vi "输入数据解析.vi"(0 "单个参数补充":dbl, 1 "从板号":dbl=1.0, 2 "主板二维码":string="BNET01", 3 "从板二维码":string="BNET01", 5 "主板引用":refnum<vi>, 7 "从板引用":refnum<vi>, 9 "主板选项":string="三级故障阀值", 11 "枚举":enum16{"主板", "从板"}(ring), 12 "快换":bool caption="快换写入") -> (4 "输出数组":dbl[][](array[numeric]), 6 "数组长度":dbl[](array[numeric]), 8 "循环次数":i32, 10 "命令":u32, 14 "名称":string[](array[string]), 15 "命令序号":u32[](array[numeric]))   [LabVIEW 2013] (continued)
                    n2574 = call "输入分辨率计算-EV05.vi"("1字节?"=FALSE, "数值"=w6626, "偏移量"=0.0, "分辨率"=0.001) -> ("低字节"=w6628:dbl, "高字节1"=w6630:dbl)  [unwired: 1 in, 5 out]
                  }
                  frame Enabled {
                    w6633 = 255 ("高字节1")
                  }
                }
                n2575 = Build Array(w6625, w6623) -> (w6624:i32[])
              }
              frame 7 {
                # "单体电压过高"
                n2576 = disable-structure shown="启用" {
                  disable-tunnel: [w6642 w6645] -> w6637
                  disable-tunnel: [w6640 w6645] -> w6635
                  disable-tunnel: w6634 -> [w6639 _]
                  frame Disabled {
                    n2577 = Unbundle By Name(w6639) -> ("单体电压过高"=w6638:dbl)
                    n2578 = call "输入分辨率计算-EV05.vi"("1字节?"=FALSE, "数值"=w6638, "偏移量"=0.0, "分辨率"=0.001) -> ("低字节"=w6640:dbl, "高字节1"=w6642:dbl)  [unwired: 1 in, 5 out]
                  }
                  frame Enabled {
                    w6645 = 255 ("高字节1")
                  }
                }
                n2579 = Build Array(w6637, w6635) -> (w6636:i32[])
              }
              frame 8 {
                # "单体电压过低"
                n2580 = disable-structure shown="启用" {
                  disable-tunnel: [w6654 w6657] -> w6649
                  disable-tunnel: [w6652 w6657] -> w6647
                  disable-tunnel: w6646 -> [w6651 _]
                  frame Enabled {
                    n2581 = Unbundle By Name(w6651) -> ("单体电压过低"=w6650:dbl)
                    n2582 = call "输入分辨率计算-EV05.vi"("1字节?"=FALSE, "数值"=w6650, "偏移量"=0.0, "分辨率"=0.001) -> ("低字节"=w6652:dbl, "高字节1"=w6654:dbl)  [unwired: 1 in, 5 out]
                  }
                  frame Disabled {
                    w6657 = 255 ("高字节1")
                  }
                }
                n2583 = Build Array(w6649, w6647) -> (w6648:dbl[])
              }
              frame 9 {
                # "充电电流过高"
                n2584 = disable-structure shown="启用" {
                  disable-tunnel: [w6666 w6669] -> w6661
                  disable-tunnel: [w6664 w6669] -> w6659
                  disable-tunnel: w6658 -> [w6663 _]
                  frame Disabled {
                    n2585 = Unbundle By Name(w6663) -> ("充电电流过高"=w6662:dbl)
                    n2586 = call "输入分辨率计算-EV05.vi"("1字节?"=FALSE, "数值"=w6662, "偏移量"=-3000.0, "分辨率"=0.1) -> ("低字节"=w6664:dbl, "高字节1"=w6666:dbl)  [unwired: 1 in, 5 out]
                  }
                  frame Enabled {
                    w6669 = 255 ("高字节1")
                  }
                }
                n2587 = Build Array(w6661, w6659) -> (w6660:i32[])
              }
              frame 10 {
                # "放电电流过高"
                n2588 = disable-structure shown="启用" {
                  disable-tunnel: [w6678 w6681] -> w6673
                  disable-tunnel: [w6676 w6681] -> w6671
                  disable-tunnel: w6670 -> [w6675 _]
                  frame Disabled {
                    n2589 = Unbundle By Name(w6675) -> ("放电电流过高"=w6674:dbl)
                    n2590 = call "输入分辨率计算-EV05.vi"("1字节?"=FALSE, "数值"=w6674, "偏移量"=-3000.0, "分辨率"=0.1) -> ("低字节"=w6676:dbl, "高字节1"=w6678:dbl)  [unwired: 1 in, 5 out]
                  }
                  frame Enabled {
                    w6681 = 255 ("高字节1")
                  }
                }
                n2591 = Build Array(w6673, w6671) -> (w6672:i32[])
              }
              frame 11 {
                # "单组温度不均衡"
                n2592 = disable-structure shown="启用" {
                  disable-tunnel: [w6688 255 ("高字节1")] -> w6684
                  disable-tunnel: w6682 -> [w6686 _]
                  frame Disabled {
                    n2593 = Unbundle By Name(w6686) -> ("单组温度不均衡"=w6685:dbl)
                    n2594 = call "输入分辨率计算-EV05.vi"("1字节?"=TRUE, "数值"=w6685, "偏移量"=0.0, "分辨率"=1.0) -> ("高字节1"=w6688:dbl)  [unwired: 1 in, 6 out]
                  }
                  frame Enabled {
                  }
                }
                n2595 = Build Array(w6684) -> (w6683:i32[])
              }
              frame 12 {
                # "SOC过高"
                n2596 = Unbundle By Name(w6696) -> ("SOC过高"=w6695:dbl)
                n2597 = call "输入分辨率计算-EV05.vi"("1字节?"=FALSE, "数值"=w6695, "偏移量"=0.0, "分辨率"=0.1) -> ("低字节"=w6697:dbl, "高字节1"=w6698:dbl)  [unwired: 1 in, 5 out]
                n2598 = call "二进制解析-8.6.vi"("索引"=4, "数值"=w6698) -> ("低位子数组"=w6701:i32[])  [unwired: 3 out]
                n2599 = call "二进制解析-8.6.vi"("索引"=4, "数值"=w6697) -> ("低位子数组"=w6693:i32[], "高位子数组"=w6700:i32[])  [unwired: 2 out]
                n2600 = Insert Into Array(array=w6701, new element=w6700) -> (w6699:i32[])  [unwired: 1 in]
                n2601 = call "数值二进制转十进制-8.6.vi"("子数组"=w6699) -> ("十进制数值"=w6694:i32)  [unwired: 4 out]
                n2602 = disable-structure shown="启用" {
                  disable-tunnel: w6694 -> [w6709 _]
                  disable-tunnel: [w6709 255 ("高字节1")] -> w6692
                  disable-tunnel: [w6708 i32[] [] ("低位子数组 26")] -> _
                  disable-tunnel: w6693 -> [w6708 _]
                  frame Disabled {
                  }
                  frame Enabled {
                  }
                }
                n2603 = Build Array(w6692, w6692) -> (w6705:i32[])
              }
              frame 13 {
                # "SOC过低"
                n2604 = Unbundle By Name(w6717) -> ("SOC过低"=w6716:dbl)
                n2605 = call "输入分辨率计算-EV05.vi"("1字节?"=FALSE, "数值"=w6716, "偏移量"=0.0, "分辨率"=0.1) -> ("低字节"=w6714:dbl, "高字节1"=w6715:dbl)  [unwired: 1 in, 5 out]
                n2606 = call "二进制解析-8.6.vi"("索引"=4, "数值"=w6715) -> ("低位子数组"=w6713:i32[])  [unwired: 3 out]
                n2607 = disable-structure shown="启用" {
                  disable-tunnel: w6714 -> [w6724 _]
                  disable-tunnel: [w6724 255 ("高字节1")] -> w6712
                  disable-tunnel: w6713 -> [w6723 _]
                  frame Disabled {
                    (unwired) i32[] [] ("低位子数组 4")
                  }
                  frame Enabled {
                  }
                }
                n2608 = Build Array(w6712, w6712) -> (w6720:i32[])
              }
              frame 14 {
                # "内阻过大"
                n2609 = disable-structure shown="启用" {
                  disable-tunnel: w6728 -> [w6733 _]
                  disable-tunnel: [w6729 255 ("高字节1")] -> w6726
                  frame Disabled {
                    n2610 = Unbundle By Name(w6733) -> ("内阻过大"=w6732:dbl)
                    n2611 = call "输入分辨率计算-EV05.vi"("1字节?"=TRUE, "数值"=w6732, "分辨率"=0.1) -> ("高字节1"=w6729:dbl)  [unwired: 2 in, 6 out]
                  }
                  frame Enabled {
                  }
                }
                n2612 = Build Array(w6726) -> (w6727:i32[])
              }
              frame 15 {
                # "极柱温度过高"
                n2613 = disable-structure shown="启用" {
                  disable-tunnel: w6737 -> [w6743 _]
                  disable-tunnel: [w6739 255 ("高字节1")] -> w6735
                  frame Disabled {
                    n2614 = Unbundle By Name(w6743) -> ("极柱温度过高"=w6742:dbl)
                    n2615 = call "输入分辨率计算-EV05.vi"("1字节?"=TRUE, "数值"=w6742, "偏移量"=-40.0, "分辨率"=1.0) -> ("高字节1"=w6739:dbl)  [unwired: 1 in, 6 out]
                  }
                  frame Enabled {
                  }
                }
                n2616 = Build Array(w6735) -> (w6736:i32[])
              }
              frame 16 {
                # "SOH过低"
                n2617 = disable-structure shown="启用" {
                  disable-tunnel: [w6760 w6768] -> w6747
                  disable-tunnel: w6746 -> [w6757 _]
                  disable-tunnel: [w6749 w6768] -> w6745
                  frame Disabled {
                    n2618 = Unbundle By Name(w6757) -> ("SOH过低"=w6756:dbl)
                    n2619 = call "输入分辨率计算-EV05.vi"("1字节?"=FALSE, "数值"=w6756, "偏移量"=0.0, "分辨率"=0.1) -> ("低字节"=w6758:dbl, "高字节1"=w6759:dbl)  [unwired: 1 in, 5 out]
                    n2620 = call "二进制解析-8.6.vi"("索引"=4, "数值"=w6759) -> ("低位子数组"=w6762:i32[])  [unwired: 3 out]
                    n2621 = call "二进制解析-8.6.vi"("索引"=4, "数值"=w6758) -> ("低位子数组"=w6751:i32[], "高位子数组"=w6761:i32[])  [unwired: 2 out]
                    n2622 = call "二进制解析-8.6.vi"("索引"=4, "数值"=0) -> ("低位子数组"=w6752:i32[])  [unwired: 3 out]
                    n2623 = Insert Into Array(array=w6762, new element=w6761) -> (w6755:i32[])  [unwired: 1 in]
                    n2624 = Insert Into Array(array=w6751, new element=w6752) -> (w6750:i32[])  [unwired: 1 in]
                    n2625 = call "数值二进制转十进制-8.6.vi"("子数组"=w6755) -> ("十进制数值"=w6760:i32)  [unwired: 4 out]
                    n2626 = call "数值二进制转十进制-8.6.vi"("子数组"=w6750) -> ("十进制数值"=w6749:i32)  [unwired: 4 out]
                  }
                  frame Enabled {
                    w6768 = 255 ("高字节1")
                  }
                }
                n2627 = Build Array(w6747, w6745) -> (w6748:i32[])
              }
            }
            n2628 = Insert Into Array(array=w6554, new element=w6555) -> (w6553:dbl[])  [unwired: 1 in]
          }
          n2629 = Build Array(w6550) -> (w6549:dbl[][])
          n2630 = Build Array("一级故障阀值") -> (w6540:string[])
        }
        frame "单体电压过低(2)" {
          n2631 = Unbundle By Name(w6774) -> ("一级故障 2"=w6775:refnum<vi>)
          n2632 = property class="Clust (严格)"(reference=w6775) -> ("Value"=w6773:T4)  [unwired: 1 in, 2 out]
          n2633 = for {
            N: 17 -> [_]
            tunnel: w6773 -> [w6785]
            shift-right: [w6782] -> w6779
            shift-left: dbl[] [] -> [w6783]
            i -> [w6786]
            n2634 = case shown="13" w6786 {
              tunnel: w6785 -> [w6787 w6798 w6809 w6819 w6829 w6839 w6851 w6863 w6875 w6887 w6899 w6911 w6925 w6946 w6957 w6966 w6975]
              tunnel: [w6788 w6799 w6810 w6820 w6830 w6841 w6853 w6865 w6877 w6889 w6901 w6912 w6934 w6949 w6956 w6965 w6977] -> w6784
              frame 0, Default {
                # "总电压过高"
                n2635 = disable-structure shown="启用" {
                  disable-tunnel: [w6794 w6797] -> w6790
                  disable-tunnel: [w6793 w6797] -> w6789
                  disable-tunnel: w6787 -> [w6792 _]
                  frame Disabled {
                    n2636 = Unbundle By Name(w6792) -> ("总电压过高"=w6791:dbl)
                    n2637 = call "输入分辨率计算-EV05.vi"("1字节?"=FALSE, "数值"=w6791, "分辨率"=0.1) -> ("低字节"=w6794:dbl, "高字节1"=w6793:dbl)  [unwired: 2 in, 5 out]
                  }
                  frame Enabled {
                    w6797 = 255 ("高字节1")
                  }
                }
                n2638 = Build Array(w6789, w6790) -> (w6788:i32[])
              }
              frame 1 {
                # "总电压过低"
                n2639 = disable-structure shown="启用" {
                  disable-tunnel: [w6805 w6808] -> w6801
                  disable-tunnel: [w6804 w6808] -> w6800
                  disable-tunnel: w6798 -> [w6803 _]
                  frame Disabled {
                    n2640 = Unbundle By Name(w6803) -> ("总电压过低"=w6802:dbl)
                    n2641 = call "输入分辨率计算-EV05.vi"("1字节?"=FALSE, "数值"=w6802, "分辨率"=0.1) -> ("低字节"=w6805:dbl, "高字节1"=w6804:dbl)  [unwired: 2 in, 5 out]
                  }
                  frame Enabled {
                    w6808 = 255 ("高字节1")
                  }
                }
                n2642 = Build Array(w6800, w6801) -> (w6799:i32[])
              }
              frame 2 {
                # "温度过高"
                n2643 = disable-structure shown="启用" {
                  disable-tunnel: [w6815 255 ("高字节1")] -> w6811
                  disable-tunnel: w6809 -> [w6813 _]
                  frame Disabled {
                    n2644 = Unbundle By Name(w6813) -> ("温度过高"=w6812:dbl)
                    n2645 = call "输入分辨率计算-EV05.vi"("1字节?"=TRUE, "数值"=w6812, "偏移量"=-40.0, "分辨率"=1.0) -> ("高字节1"=w6815:dbl)  [unwired: 1 in, 6 out]
                  }
                  frame Enabled {
                  }
                }
                n2646 = Build Array(w6811) -> (w6810:i32[])
              }
              frame 3 {
                # "温度过低"
                n2647 = disable-structure shown="启用" {
                  disable-tunnel: [w6825 255 ("高字节1")] -> w6821
                  disable-tunnel: w6819 -> [w6823 _]
                  frame Disabled {
                    n2648 = Unbundle By Name(w6823) -> ("温度过低"=w6822:dbl)
                    n2649 = call "输入分辨率计算-EV05.vi"("1字节?"=TRUE, "数值"=w6822, "偏移量"=-40.0, "分辨率"=1.0) -> ("高字节1"=w6825:dbl)  [unwired: 1 in, 6 out]
                  }
                  frame Enabled {
                  }
                }
                n2650 = Build Array(w6821) -> (w6820:i32[])
              }
              frame 4 {
                # "整组温度不均衡"
                n2651 = disable-structure shown="启用" {
                  disable-tunnel: [w6835 255 ("高字节1")] -> w6831
                  disable-tunnel: w6829 -> [w6833 _]
                  frame Disabled {
                    n2652 = Unbundle By Name(w6833) -> ("整组温度不均衡"=w6832:dbl)
                    n2653 = call "输入分辨率计算-EV05.vi"("1字节?"=TRUE, "数值"=w6832, "偏移量"=0.0, "分辨率"=1.0) -> ("高字节1"=w6835:dbl)  [unwired: 1 in, 6 out]
                  }
                  frame Enabled {
                  }
                }
                n2654 = Build Array(w6831) -> (w6830:i32[])
              }
              frame 5 {
                # "单组电压不均衡"
                n2655 = disable-structure shown="启用" {
                  disable-tunnel: [w6847 w6850] -> w6842
                  disable-tunnel: [w6845 w6850] -> w6840
                  disable-tunnel: w6839 -> [w6844 _]
                  frame Disabled {
                    n2656 = Unbundle By Name(w6844) -> ("单组电压不均衡"=w6843:dbl)
                    n2657 = call "输入分辨率计算-EV05.vi"("1字节?"=FALSE, "数值"=w6843, "偏移量"=0.0, "分辨率"=0.001) -> ("低字节"=w6845:dbl, "高字节1"=w6847:dbl)  [unwired: 1 in, 5 out]
                  }
                  frame Enabled {
                    w6850 = 255 ("高字节1")
                  }
                }
                n2658 = Build Array(w6842, w6840) -> (w6841:i32[])
              }
              frame 6 {
                # "整组电压不均衡"
                n2659 = disable-structure shown="启用" {
                  disable-tunnel: [w6859 w6862] -> w6854
                  disable-tunnel: [w6857 w6862] -> w6852
                  disable-tunnel: w6851 -> [w6856 _]
                  frame Disabled {
                    n2660 = Unbundle By Name(w6856) -> ("整组电压不均衡"=w6855:dbl)
                    n2661 = call "输入分辨率计算-EV05.vi"("1字节?"=FALSE, "数值"=w6855, "偏移量"=0.0, "分辨率"=0.001) -> ("低字节"=w6857:dbl, "高字节1"=w6859:dbl)  [unwired: 1 in, 5 out]
                  }
                  frame Enabled {
                    w6862 = 255 ("高字节1")
                  }
                }
                n2662 = Build Array(w6854, w6852) -> (w6853:i32[])
              }
              frame 7 {
                # "单体电压过高"
                n2663 = disable-structure shown="启用" {
                  disable-tunnel: [w6871 w6874] -> w6866
                  disable-tunnel: [w6869 w6874] -> w6864
                  disable-tunnel: w6863 -> [w6868 _]
                  frame Disabled {
                    n2664 = Unbundle By Name(w6868) -> ("单体电压过高"=w6867:dbl)
                    n2665 = call "输入分辨率计算-EV05.vi"("1字节?"=FALSE, "数值"=w6867, "偏移量"=0.0, "分辨率"=0.001) -> ("低字节"=w6869:dbl, "高字节1"=w6871:dbl)  [unwired: 1 in, 5 out]
                  }
                  frame Enabled {
                    w6874 = 255 ("高字节1")
                  }
                }
                n2666 = Build Array(w6866, w6864) -> (w6865:i32[])
              }
              frame 8 {
                # "单体电压过低"
                n2667 = disable-structure shown="启用" {
                  disable-tunnel: [w6883 w6886] -> w6878
                  disable-tunnel: [w6881 w6886] -> w6876
                  disable-tunnel: w6875 -> [w6880 _]
                  frame Enabled {
                    n2668 = Unbundle By Name(w6880) -> ("单体电压过低"=w6879:dbl)
                    n2669 = call "输入分辨率计算-EV05.vi"("1字节?"=FALSE, "数值"=w6879, "偏移量"=0.0, "分辨率"=0.001) -> ("低字节"=w6881:dbl, "高字节1"=w6883:dbl)  [unwired: 1 in, 5 out]
                  }
                  frame Disabled {
                    w6886 = 255 ("高字节1")
                  }
                }
                n2670 = Build Array(w6878, w6876) -> (w6877:dbl[])
              }
              frame 9 {
                # "充电电流过高"
                n2671 = disable-structure shown="启用" {
                  disable-tunnel: [w6895 w6898] -> w6890
                  disable-tunnel: [w6893 w6898] -> w6888
                  disable-tunnel: w6887 -> [w6892 _]
                  frame Disabled {
                    n2672 = Unbundle By Name(w6892) -> ("充电电流过高"=w6891:dbl)
                    n2673 = call "输入分辨率计算-EV05.vi"("1字节?"=FALSE, "数值"=w6891, "偏移量"=-3000.0, "分辨率"=0.1) -> ("低字节"=w6893:dbl, "高字节1"=w6895:dbl)  [unwired: 1 in, 5 out]
                  }
                  frame Enabled {
                    w6898 = 255 ("高字节1")
                  }
                }
                n2674 = Build Array(w6890, w6888) -> (w6889:i32[])
              }
              frame 10 {
                # "放电电流过高"
                n2675 = disable-structure shown="启用" {
                  disable-tunnel: [w6907 w6910] -> w6902
                  disable-tunnel: [w6905 w6910] -> w6900
                  disable-tunnel: w6899 -> [w6904 _]
                  frame Disabled {
                    n2676 = Unbundle By Name(w6904) -> ("放电电流过高"=w6903:dbl)
                    n2677 = call "输入分辨率计算-EV05.vi"("1字节?"=FALSE, "数值"=w6903, "偏移量"=-3000.0, "分辨率"=0.1) -> ("低字节"=w6905:dbl, "高字节1"=w6907:dbl)  [unwired: 1 in, 5 out]
                  }
                  frame Enabled {
                    w6910 = 255 ("高字节1")
                  }
                }
                n2678 = Build Array(w6902, w6900) -> (w6901:i32[])
              }
              frame 11 {
                # "单组温度不均衡"
                n2679 = disable-structure shown="启用" {
                  disable-tunnel: [w6917 255 ("高字节1")] -> w6913
                  disable-tunnel: w6911 -> [w6915 _]
                  frame Disabled {
                    n2680 = Unbundle By Name(w6915) -> ("单组温度不均衡"=w6914:dbl)
                    n2681 = call "输入分辨率计算-EV05.vi"("1字节?"=TRUE, "数值"=w6914, "偏移量"=0.0, "分辨率"=1.0) -> ("高字节1"=w6917:dbl)  [unwired: 1 in, 6 out]
                  }
                  frame Enabled {
                  }
                }
                n2682 = Build Array(w6913) -> (w6912:i32[])
              }
              frame 12 {
                # "SOC过高"
                n2683 = Unbundle By Name(w6925) -> ("SOC过高"=w6924:dbl)
                n2684 = call "输入分辨率计算-EV05.vi"("1字节?"=FALSE, "数值"=w6924, "偏移量"=0.0, "分辨率"=0.1) -> ("低字节"=w6926:dbl, "高字节1"=w6927:dbl)  [unwired: 1 in, 5 out]
                n2685 = call "二进制解析-8.6.vi"("索引"=4, "数值"=w6927) -> ("低位子数组"=w6930:i32[])  [unwired: 3 out]
                n2686 = call "二进制解析-8.6.vi"("索引"=4, "数值"=w6926) -> ("低位子数组"=w6922:i32[], "高位子数组"=w6929:i32[])  [unwired: 2 out]
                n2687 = Insert Into Array(array=w6930, new element=w6929) -> (w6928:i32[])  [unwired: 1 in]
                n2688 = call "数值二进制转十进制-8.6.vi"("子数组"=w6928) -> ("十进制数值"=w6923:i32)  [unwired: 4 out]
                n2689 = disable-structure shown="启用" {
                  disable-tunnel: w6923 -> [w6938 _]
                  disable-tunnel: [w6938 255 ("高字节1")] -> w6921
                  disable-tunnel: [w6937 i32[] [] ("低位子数组 26")] -> _
                  disable-tunnel: w6922 -> [w6937 _]
                  frame Disabled {
                  }
                  frame Enabled {
                  }
                }
                n2690 = Build Array(w6921, w6921) -> (w6934:i32[])
              }
              frame 13 {
                # "SOC过低"
                n2691 = Unbundle By Name(w6946) -> ("SOC过低"=w6945:dbl)
                n2692 = call "输入分辨率计算-EV05.vi"("1字节?"=FALSE, "数值"=w6945, "偏移量"=0.0, "分辨率"=0.1) -> ("低字节"=w6943:dbl, "高字节1"=w6944:dbl)  [unwired: 1 in, 5 out]
                n2693 = call "二进制解析-8.6.vi"("索引"=4, "数值"=w6944) -> ("低位子数组"=w6942:i32[])  [unwired: 3 out]
                n2694 = disable-structure shown="启用" {
                  disable-tunnel: w6943 -> [w6953 _]
                  disable-tunnel: [w6953 255 ("高字节1")] -> w6941
                  disable-tunnel: w6942 -> [w6952 _]
                  frame Disabled {
                    (unwired) i32[] [] ("低位子数组 4")
                  }
                  frame Enabled {
                  }
                }
                n2695 = Build Array(w6941, w6941) -> (w6949:i32[])
              }
              frame 14 {
                # "内阻过大"
                n2696 = disable-structure shown="启用" {
                  disable-tunnel: w6957 -> [w6962 _]
                  disable-tunnel: [w6958 255 ("高字节1")] -> w6955
                  frame Disabled {
                    n2697 = Unbundle By Name(w6962) -> ("内阻过大"=w6961:dbl)
                    n2698 = call "输入分辨率计算-EV05.vi"("1字节?"=TRUE, "数值"=w6961, "分辨率"=0.1) -> ("高字节1"=w6958:dbl)  [unwired: 2 in, 6 out]
                  }
                  frame Enabled {
                  }
                }
                n2699 = Build Array(w6955) -> (w6956:i32[])
              }
              frame 15 {
                # "极柱温度过高"
                n2700 = disable-structure shown="启用" {
                  disable-tunnel: w6966 -> [w6972 _]
                  disable-tunnel: [w6968 255 ("高字节1")] -> w6964
                  frame Disabled {
                    n2701 = Unbundle By Name(w6972) -> ("极柱温度过高"=w6971:dbl)
                    n2702 = call "输入分辨率计算-EV05.vi"("1字节?"=TRUE, "数值"=w6971, "偏移量"=-40.0, "分辨率"=1.0) -> ("高字节1"=w6968:dbl)  [unwired: 1 in, 6 out]
                  }
                  frame Enabled {
                  }
                }
                n2703 = Build Array(w6964) -> (w6965:i32[])
              }
              frame 16 {
                # "SOH过低"
                n2704 = disable-structure shown="启用" {
                  disable-tunnel: [w6989 w6997] -> w6976
                  disable-tunnel: w6975 -> [w6986 _]
                  disable-tunnel: [w6978 w6997] -> w6974
                  frame Disabled {
                    n2705 = Unbundle By Name(w6986) -> ("SOH过低"=w6985:dbl)
                    n2706 = call "输入分辨率计算-EV05.vi"("1字节?"=FALSE, "数值"=w6985, "偏移量"=0.0, "分辨率"=0.1) -> ("低字节"=w6987:dbl, "高字节1"=w6988:dbl)  [unwired: 1 in, 5 out]
                    n2707 = call "二进制解析-8.6.vi"("索引"=4, "数值"=w6988) -> ("低位子数组"=w6991:i32[])  [unwired: 3 out]
                    n2708 = call "二进制解析-8.6.vi"("索引"=4, "数值"=w6987) -> ("低位子数组"=w6980:i32[], "高位子数组"=w6990:i32[])  [unwired: 2 out]
                    n2709 = call "二进制解析-8.6.vi"("索引"=4, "数值"=0) -> ("低位子数组"=w6981:i32[])  [unwired: 3 out]
                    n2710 = Insert Into Array(array=w6991, new element=w6990) -> (w6984:i32[])  [unwired: 1 in]
                    n2711 = Insert Into Array(array=w6980, new element=w6981) -> (w6979:i32[])  [unwired: 1 in]
                    n2712 = call "数值二进制转十进制-8.6.vi"("子数组"=w6984) -> ("十进制数值"=w6989:i32)  [unwired: 4 out]
                    n2713 = call "数值二进制转十进制-8.6.vi"("子数组"=w6979) -> ("十进制数值"=w6978:i32)  [unwired: 4 out]
                  }
                  frame Enabled {
                    w6997 = 255 ("高字节1")
                  }
                }
                n2714 = Build Array(w6976, w6974) -> (w6977:i32[])
              }
            }
            n2715 = Insert Into Array(array=w6783, new element=w6784) -> (w6782:dbl[])  [unwired: 1 in]
          }
          n2716 = Build Array(w6779) -> (w6778:dbl[][])
          n2717 = Build Array("二级故障阀值") -> (w6769:string[])
        }
        frame "单体电压过低(3)" {
          n2718 = Unbundle By Name(w7003) -> ("一级故障 3"=w7004:refnum<vi>)
          n2719 = property class="Clust (严格)"(reference=w7004) -> ("Value"=w7002:T4)  [unwired: 1 in, 2 out]
          n2720 = for {
            N: 17 -> [_]
            tunnel: w7002 -> [w7014]
            shift-right: [w7011] -> w7008
            shift-left: dbl[] [] -> [w7012]
            i -> [w7015]
            n2721 = case shown="13" w7015 {
              tunnel: w7014 -> [w7016 w7027 w7038 w7048 w7058 w7068 w7080 w7092 w7104 w7116 w7128 w7140 w7154 w7175 w7186 w7195 w7204]
              tunnel: [w7017 w7028 w7039 w7049 w7059 w7070 w7082 w7094 w7106 w7118 w7130 w7141 w7163 w7178 w7185 w7194 w7206] -> w7013
              frame 0, Default {
                # "总电压过高"
                n2722 = disable-structure shown="启用" {
                  disable-tunnel: [w7023 w7026] -> w7019
                  disable-tunnel: [w7022 w7026] -> w7018
                  disable-tunnel: w7016 -> [w7021 _]
                  frame Disabled {
                    n2723 = Unbundle By Name(w7021) -> ("总电压过高"=w7020:dbl)
                    n2724 = call "输入分辨率计算-EV05.vi"("1字节?"=FALSE, "数值"=w7020, "分辨率"=0.1) -> ("低字节"=w7023:dbl, "高字节1"=w7022:dbl)  [unwired: 2 in, 5 out]
                  }
                  frame Enabled {
                    w7026 = 255 ("高字节1")
                  }
                }
                n2725 = Build Array(w7018, w7019) -> (w7017:i32[])
              }
              frame 1 {
                # "总电压过低"
                n2726 = disable-structure shown="启用" {
                  disable-tunnel: [w7034 w7037] -> w7030
                  disable-tunnel: [w7033 w7037] -> w7029
                  disable-tunnel: w7027 -> [w7032 _]
                  frame Disabled {
                    n2727 = Unbundle By Name(w7032) -> ("总电压过低"=w7031:dbl)
                    n2728 = call "输入分辨率计算-EV05.vi"("1字节?"=FALSE, "数值"=w7031, "分辨率"=0.1) -> ("低字节"=w7034:dbl, "高字节1"=w7033:dbl)  [unwired: 2 in, 5 out]
                  }
                  frame Enabled {
                    w7037 = 255 ("高字节1")
                  }
                }
                n2729 = Build Array(w7029, w7030) -> (w7028:i32[])
              }
              frame 2 {
                # "温度过高"
                n2730 = disable-structure shown="启用" {
                  disable-tunnel: [w7044 255 ("高字节1")] -> w7040
                  disable-tunnel: w7038 -> [w7042 _]
                  frame Disabled {
                    n2731 = Unbundle By Name(w7042) -> ("温度过高"=w7041:dbl)
                    n2732 = call "输入分辨率计算-EV05.vi"("1字节?"=TRUE, "数值"=w7041, "偏移量"=-40.0, "分辨率"=1.0) -> ("高字节1"=w7044:dbl)  [unwired: 1 in, 6 out]
                  }
                  frame Enabled {
                  }
                }
                n2733 = Build Array(w7040) -> (w7039:i32[])
              }
              frame 3 {
                # "温度过低"
                n2734 = disable-structure shown="启用" {
                  disable-tunnel: [w7054 255 ("高字节1")] -> w7050
                  disable-tunnel: w7048 -> [w7052 _]
                  frame Disabled {
                    n2735 = Unbundle By Name(w7052) -> ("温度过低"=w7051:dbl)
                    n2736 = call "输入分辨率计算-EV05.vi"("1字节?"=TRUE, "数值"=w7051, "偏移量"=-40.0, "分辨率"=1.0) -> ("高字节1"=w7054:dbl)  [unwired: 1 in, 6 out]
                  }
                  frame Enabled {
                  }
                }
                n2737 = Build Array(w7050) -> (w7049:i32[])
              }
              frame 4 {
                # "整组温度不均衡"
                n2738 = disable-structure shown="启用" {
                  disable-tunnel: [w7064 255 ("高字节1")] -> w7060
                  disable-tunnel: w7058 -> [w7062 _]
                  frame Disabled {
                    n2739 = Unbundle By Name(w7062) -> ("整组温度不均衡"=w7061:dbl)
                    n2740 = call "输入分辨率计算-EV05.vi"("1字节?"=TRUE, "数值"=w7061, "偏移量"=0.0, "分辨率"=1.0) -> ("高字节1"=w7064:dbl)  [unwired: 1 in, 6 out]
                  }
                  frame Enabled {
                  }
                }
                n2741 = Build Array(w7060) -> (w7059:i32[])
              }
              frame 5 {
                # "单组电压不均衡"
                n2742 = disable-structure shown="启用" {
                  disable-tunnel: [w7076 w7079] -> w7071
                  disable-tunnel: [w7074 w7079] -> w7069
                  disable-tunnel: w7068 -> [w7073 _]
                  frame Disabled {
                    n2743 = Unbundle By Name(w7073) -> ("单组电压不均衡"=w7072:dbl)
                    n2744 = call "输入分辨率计算-EV05.vi"("1字节?"=FALSE, "数值"=w7072, "偏移量"=0.0, "分辨率"=0.001) -> ("低字节"=w7074:dbl, "高字节1"=w7076:dbl)  [unwired: 1 in, 5 out]
                  }
                  frame Enabled {
                    w7079 = 255 ("高字节1")
                  }
                }
                n2745 = Build Array(w7071, w7069) -> (w7070:i32[])
              }
              frame 6 {
                # "整组电压不均衡"
                n2746 = disable-structure shown="启用" {
                  disable-tunnel: [w7088 w7091] -> w7083
                  disable-tunnel: [w7086 w7091] -> w7081
                  disable-tunnel: w7080 -> [w7085 _]
                  frame Disabled {
                    n2747 = Unbundle By Name(w7085) -> ("整组电压不均衡"=w7084:dbl)
                    n2748 = call "输入分辨率计算-EV05.vi"("1字节?"=FALSE, "数值"=w7084, "偏移量"=0.0, "分辨率"=0.001) -> ("低字节"=w7086:dbl, "高字节1"=w7088:dbl)  [unwired: 1 in, 5 out]
                  }
                  frame Enabled {
                    w7091 = 255 ("高字节1")
                  }
                }
                n2749 = Build Array(w7083, w7081) -> (w7082:i32[])
              }
              frame 7 {
                # "单体电压过高"
                n2750 = disable-structure shown="启用" {
                  disable-tunnel: [w7100 w7103] -> w7095
                  disable-tunnel: [w7098 w7103] -> w7093
                  disable-tunnel: w7092 -> [w7097 _]
                  frame Disabled {
                    n2751 = Unbundle By Name(w7097) -> ("单体电压过高"=w7096:dbl)
                    n2752 = call "输入分辨率计算-EV05.vi"("1字节?"=FALSE, "数值"=w7096, "偏移量"=0.0, "分辨率"=0.001) -> ("低字节"=w7098:dbl, "高字节1"=w7100:dbl)  [unwired: 1 in, 5 out]
                  }
                  frame Enabled {
                    w7103 = 255 ("高字节1")
                  }
                }
                n2753 = Build Array(w7095, w7093) -> (w7094:i32[])
              }
              frame 8 {
                # "单体电压过低"
                n2754 = disable-structure shown="启用" {
                  disable-tunnel: [w7112 w7115] -> w7107
                  disable-tunnel: [w7110 w7115] -> w7105
                  disable-tunnel: w7104 -> [w7109 _]
                  frame Enabled {
                    n2755 = Unbundle By Name(w7109) -> ("单体电压过低"=w7108:dbl)
                    n2756 = call "输入分辨率计算-EV05.vi"("1字节?"=FALSE, "数值"=w7108, "偏移量"=0.0, "分辨率"=0.001) -> ("低字节"=w7110:dbl, "高字节1"=w7112:dbl)  [unwired: 1 in, 5 out]
                  }
                  frame Disabled {
                    w7115 = 255 ("高字节1")
                  }
                }
                n2757 = Build Array(w7107, w7105) -> (w7106:dbl[])
              }
              frame 9 {
                # "充电电流过高"
                n2758 = disable-structure shown="启用" {
                  disable-tunnel: [w7124 w7127] -> w7119
                  disable-tunnel: [w7122 w7127] -> w7117
                  disable-tunnel: w7116 -> [w7121 _]
                  frame Disabled {
                    n2759 = Unbundle By Name(w7121) -> ("充电电流过高"=w7120:dbl)
                    n2760 = call "输入分辨率计算-EV05.vi"("1字节?"=FALSE, "数值"=w7120, "偏移量"=-3000.0, "分辨率"=0.1) -> ("低字节"=w7122:dbl, "高字节1"=w7124:dbl)  [unwired: 1 in, 5 out]
                  }
                  frame Enabled {
                    w7127 = 255 ("高字节1")
                  }
                }
                n2761 = Build Array(w7119, w7117) -> (w7118:i32[])
              }
              frame 10 {
                # "放电电流过高"
                n2762 = disable-structure shown="启用" {
                  disable-tunnel: [w7136 w7139] -> w7131
                  disable-tunnel: [w7134 w7139] -> w7129
                  disable-tunnel: w7128 -> [w7133 _]
                  frame Disabled {
                    n2763 = Unbundle By Name(w7133) -> ("放电电流过高"=w7132:dbl)
                    n2764 = call "输入分辨率计算-EV05.vi"("1字节?"=FALSE, "数值"=w7132, "偏移量"=-3000.0, "分辨率"=0.1) -> ("低字节"=w7134:dbl, "高字节1"=w7136:dbl)  [unwired: 1 in, 5 out]
                  }
                  frame Enabled {
                    w7139 = 255 ("高字节1")
                  }
                }
                n2765 = Build Array(w7131, w7129) -> (w7130:i32[])
              }
              frame 11 {
                # "单组温度不均衡"
                n2766 = disable-structure shown="启用" {
                  disable-tunnel: [w7146 255 ("高字节1")] -> w7142
                  disable-tunnel: w7140 -> [w7144 _]
                  frame Disabled {
                    n2767 = Unbundle By Name(w7144) -> ("单组温度不均衡"=w7143:dbl)
                    n2768 = call "输入分辨率计算-EV05.vi"("1字节?"=TRUE, "数值"=w7143, "偏移量"=0.0, "分辨率"=1.0) -> ("高字节1"=w7146:dbl)  [unwired: 1 in, 6 out]
                  }
                  frame Enabled {
                  }
                }
                n2769 = Build Array(w7142) -> (w7141:i32[])
              }
              frame 12 {
                # "SOC过高"
                n2770 = Unbundle By Name(w7154) -> ("SOC过高"=w7153:dbl)
                n2771 = call "输入分辨率计算-EV05.vi"("1字节?"=FALSE, "数值"=w7153, "偏移量"=0.0, "分辨率"=0.1) -> ("低字节"=w7155:dbl, "高字节1"=w7156:dbl)  [unwired: 1 in, 5 out]
                n2772 = call "二进制解析-8.6.vi"("索引"=4, "数值"=w7156) -> ("低位子数组"=w7159:i32[])  [unwired: 3 out]
                n2773 = call "二进制解析-8.6.vi"("索引"=4, "数值"=w7155) -> ("低位子数组"=w7151:i32[], "高位子数组"=w7158:i32[])  [unwired: 2 out]
                n2774 = Insert Into Array(array=w7159, new element=w7158) -> (w7157:i32[])  [unwired: 1 in]
                n2775 = call "数值二进制转十进制-8.6.vi"("子数组"=w7157) -> ("十进制数值"=w7152:i32)  [unwired: 4 out]
                n2776 = disable-structure shown="启用" {
                  disable-tunnel: w7152 -> [w7167 _]
                  disable-tunnel: [w7167 255 ("高字节1")] -> w7150
                  disable-tunnel: [w7166 i32[] [] ("低位子数组 26")] -> _
                  disable-tunnel: w7151 -> [w7166 _]
                  frame Disabled {
                  }
                  frame Enabled {
                  }
                }
                n2777 = Build Array(w7150, w7150) -> (w7163:i32[])
              }
              frame 13 {
                # "SOC过低"
                n2778 = Unbundle By Name(w7175) -> ("SOC过低"=w7174:dbl)
                n2779 = call "输入分辨率计算-EV05.vi"("1字节?"=FALSE, "数值"=w7174, "偏移量"=0.0, "分辨率"=0.1) -> ("低字节"=w7172:dbl, "高字节1"=w7173:dbl)  [unwired: 1 in, 5 out]
                n2780 = call "二进制解析-8.6.vi"("索引"=4, "数值"=w7173) -> ("低位子数组"=w7171:i32[])  [unwired: 3 out]
                n2781 = disable-structure shown="启用" {
                  disable-tunnel: w7172 -> [w7182 _]
                  disable-tunnel: [w7182 255 ("高字节1")] -> w7170
                  disable-tunnel: w7171 -> [w7181 _]
                  frame Disabled {
                    (unwired) i32[] [] ("低位子数组 4")
                  }
                  frame Enabled {
                  }
                }
                n2782 = Build Array(w7170, w7170) -> (w7178:i32[])
              }
              frame 14 {
                # "内阻过大"
                n2783 = disable-structure shown="启用" {
                  disable-tunnel: w7186 -> [w7191 _]
                  disable-tunnel: [w7187 255 ("高字节1")] -> w7184
                  frame Disabled {
                    n2784 = Unbundle By Name(w7191) -> ("内阻过大"=w7190:dbl)
                    n2785 = call "输入分辨率计算-EV05.vi"("1字节?"=TRUE, "数值"=w7190, "分辨率"=0.1) -> ("高字节1"=w7187:dbl)  [unwired: 2 in, 6 out]
                  }
                  frame Enabled {
                  }
                }
                n2786 = Build Array(w7184) -> (w7185:i32[])
              }
              frame 15 {
                # "极柱温度过高"
                n2787 = disable-structure shown="启用" {
                  disable-tunnel: w7195 -> [w7201 _]
                  disable-tunnel: [w7197 255 ("高字节1")] -> w7193
                  frame Disabled {
                    n2788 = Unbundle By Name(w7201) -> ("极柱温度过高"=w7200:dbl)
                    n2789 = call "输入分辨率计算-EV05.vi"("1字节?"=TRUE, "数值"=w7200, "偏移量"=-40.0, "分辨率"=1.0) -> ("高字节1"=w7197:dbl)  [unwired: 1 in, 6 out]
                  }
                  frame Enabled {
                  }
                }
                n2790 = Build Array(w7193) -> (w7194:i32[])
              }
              frame 16 {
                # "SOH过低"
                n2791 = disable-structure shown="启用" {
                  disable-tunnel: [w7218 w7226] -> w7205
                  disable-tunnel: w7204 -> [w7215 _]
                  disable-tunnel: [w7207 w7226] -> w7203
                  frame Disabled {
                    n2792 = Unbundle By Name(w7215) -> ("SOH过低"=w7214:dbl)
                    n2793 = call "输入分辨率计算-EV05.vi"("1字节?"=FALSE, "数值"=w7214, "偏移量"=0.0, "分辨率"=0.1) -> ("低字节"=w7216:dbl, "高字节1"=w7217:dbl)  [unwired: 1 in, 5 out]
                    n2794 = call "二进制解析-8.6.vi"("索引"=4, "数值"=w7217) -> ("低位子数组"=w7220:i32[])  [unwired: 3 out]
                    n2795 = call "二进制解析-8.6.vi"("索引"=4, "数值"=w7216) -> ("低位子数组"=w7209:i32[], "高位子数组"=w7219:i32[])  [unwired: 2 out]
                    n2796 = call "二进制解析-8.6.vi"("索引"=4, "数值"=0) -> ("低位子数组"=w7210:i32[])  [unwired: 3 out]
                    n2797 = Insert Into Array(array=w7220, new element=w7219) -> (w7213:i32[])  [unwired: 1 in]
                    n2798 = Insert Into Array(array=w7209, new element=w7210) -> (w7208:i32[])  [unwired: 1 in]
                    n2799 = call "数值二进制转十进制-8.6.vi"("子数组"=w7213) -> ("十进制数值"=w7218:i32)  [unwired: 4 out]
                    n2800 = call "数值二进制转十进制-8.6.vi"("子数组"=w7208) -> ("十进制数值"=w7207:i32)  [unwired: 4 out]
                  }
                  frame Enabled {
                    w7226 = 255 ("高字节1")
                  }
                }
                n2801 = Build Array(w7205, w7203) -> (w7206:i32[])
              }
            }
            n2802 = Insert Into Array(array=w7012, new element=w7013) -> (w7011:dbl[])  [unwired: 1 in]
          }
          n2803 = Build Array(w7008) -> (w7007:dbl[][])
          n2804 = Build Array("三级故障阀值") -> (w6998:string[])
        }
        frame "充电电流过高" {
          n2805 = Unbundle By Name(w7232) -> ("一级故障"=w7233:refnum<vi>)
          n2806 = property class="Clust (严格)"(reference=w7233) -> ("Value"=w7231:T4)  [unwired: 1 in, 2 out]
          n2807 = for {
            N: 17 -> [_]
            tunnel: w7231 -> [w7243]
            shift-right: [w7240] -> w7237
            shift-left: dbl[] [] -> [w7241]
            i -> [w7244]
            n2808 = case shown="13" w7244 {
              tunnel: w7243 -> [w7245 w7256 w7267 w7277 w7287 w7297 w7309 w7321 w7333 w7345 w7357 w7369 w7383 w7404 w7416 w7425 w7434]
              tunnel: [w7246 w7257 w7268 w7278 w7288 w7299 w7311 w7323 w7335 w7347 w7359 w7370 w7392 w7407 w7415 w7424 w7436] -> w7242
              frame 0, Default {
                # "总电压过高"
                n2809 = disable-structure shown="启用" {
                  disable-tunnel: [w7252 w7255] -> w7248
                  disable-tunnel: [w7251 w7255] -> w7247
                  disable-tunnel: w7245 -> [w7250 _]
                  frame Disabled {
                    n2810 = Unbundle By Name(w7250) -> ("总电压过高"=w7249:dbl)
                    n2811 = call "输入分辨率计算-EV05.vi"("1字节?"=FALSE, "数值"=w7249, "分辨率"=0.1) -> ("低字节"=w7252:dbl, "高字节1"=w7251:dbl)  [unwired: 2 in, 5 out]
                  }
                  frame Enabled {
                    w7255 = 255 ("高字节1")
                  }
                }
                n2812 = Build Array(w7247, w7248) -> (w7246:i32[])
              }
              frame 1 {
                # "总电压过低"
                n2813 = disable-structure shown="启用" {
                  disable-tunnel: [w7263 w7266] -> w7259
                  disable-tunnel: [w7262 w7266] -> w7258
                  disable-tunnel: w7256 -> [w7261 _]
                  frame Disabled {
                    n2814 = Unbundle By Name(w7261) -> ("总电压过低"=w7260:dbl)
                    n2815 = call "输入分辨率计算-EV05.vi"("1字节?"=FALSE, "数值"=w7260, "分辨率"=0.1) -> ("低字节"=w7263:dbl, "高字节1"=w7262:dbl)  [unwired: 2 in, 5 out]
                  }
                  frame Enabled {
                    w7266 = 255 ("高字节1")
                  }
                }
                n2816 = Build Array(w7258, w7259) -> (w7257:i32[])
              }
              frame 2 {
                # "温度过高"
                n2817 = disable-structure shown="启用" {
                  disable-tunnel: [w7273 255 ("高字节1")] -> w7269
                  disable-tunnel: w7267 -> [w7271 _]
                  frame Disabled {
                    n2818 = Unbundle By Name(w7271) -> ("温度过高"=w7270:dbl)
                    n2819 = call "输入分辨率计算-EV05.vi"("1字节?"=TRUE, "数值"=w7270, "偏移量"=-40.0, "分辨率"=1.0) -> ("高字节1"=w7273:dbl)  [unwired: 1 in, 6 out]
                  }
                  frame Enabled {
                  }
                }
                n2820 = Build Array(w7269) -> (w7268:i32[])
              }
              frame 3 {
                # "温度过低"
                n2821 = disable-structure shown="启用" {
                  disable-tunnel: [w7283 255 ("高字节1")] -> w7279
                  disable-tunnel: w7277 -> [w7281 _]
                  frame Disabled {
                    n2822 = Unbundle By Name(w7281) -> ("温度过低"=w7280:dbl)
                    n2823 = call "输入分辨率计算-EV05.vi"("1字节?"=TRUE, "数值"=w7280, "偏移量"=-40.0, "分辨率"=1.0) -> ("高字节1"=w7283:dbl)  [unwired: 1 in, 6 out]
                  }
                  frame Enabled {
                  }
                }
                n2824 = Build Array(w7279) -> (w7278:i32[])
              }
              frame 4 {
                # "整组温度不均衡"
                n2825 = disable-structure shown="启用" {
                  disable-tunnel: [w7293 255 ("高字节1")] -> w7289
                  disable-tunnel: w7287 -> [w7291 _]
                  frame Disabled {
                    n2826 = Unbundle By Name(w7291) -> ("整组温度不均衡"=w7290:dbl)
                    n2827 = call "输入分辨率计算-EV05.vi"("1字节?"=TRUE, "数值"=w7290, "偏移量"=0.0, "分辨率"=1.0) -> ("高字节1"=w7293:dbl)  [unwired: 1 in, 6 out]
                  }
                  frame Enabled {
                  }
                }
                n2828 = Build Array(w7289) -> (w7288:i32[])
              }
              frame 5 {
                # "单组电压不均衡"
                n2829 = disable-structure shown="启用" {
                  disable-tunnel: [w7305 w7308] -> w7300
                  disable-tunnel: [w7303 w7308] -> w7298
                  disable-tunnel: w7297 -> [w7302 _]
                  frame Disabled {
                    n2830 = Unbundle By Name(w7302) -> ("单组电压不均衡"=w7301:dbl)
                    n2831 = call "输入分辨率计算-EV05.vi"("1字节?"=FALSE, "数值"=w7301, "偏移量"=0.0, "分辨率"=0.001) -> ("低字节"=w7303:dbl, "高字节1"=w7305:dbl)  [unwired: 1 in, 5 out]
                  }
                  frame Enabled {
                    w7308 = 255 ("高字节1")
                  }
                }
                n2832 = Build Array(w7300, w7298) -> (w7299:i32[])
              }
              frame 6 {
                # "整组电压不均衡"
                n2833 = disable-structure shown="启用" {
                  disable-tunnel: [w7317 w7320] -> w7312
                  disable-tunnel: [w7315 w7320] -> w7310
                  disable-tunnel: w7309 -> [w7314 _]
                  frame Disabled {
                    n2834 = Unbundle By Name(w7314) -> ("整组电压不均衡"=w7313:dbl)
                    n2835 = call "输入分辨率计算-EV05.vi"("1字节?"=FALSE, "数值"=w7313, "偏移量"=0.0, "分辨率"=0.001) -> ("低字节"=w7315:dbl, "高字节1"=w7317:dbl)  [unwired: 1 in, 5 out]
                  }
                  frame Enabled {
                    w7320 = 255 ("高字节1")
                  }
                }
                n2836 = Build Array(w7312, w7310) -> (w7311:i32[])
              }
              frame 7 {
                # "单体电压过高"
                n2837 = disable-structure shown="启用" {
                  disable-tunnel: [w7329 w7332] -> w7324
                  disable-tunnel: [w7327 w7332] -> w7322
                  disable-tunnel: w7321 -> [w7326 _]
                  frame Disabled {
                    n2838 = Unbundle By Name(w7326) -> ("单体电压过高"=w7325:dbl)
                    n2839 = call "输入分辨率计算-EV05.vi"("1字节?"=FALSE, "数值"=w7325, "偏移量"=0.0, "分辨率"=0.001) -> ("低字节"=w7327:dbl, "高字节1"=w7329:dbl)  [unwired: 1 in, 5 out]
                  }
                  frame Enabled {
                    w7332 = 255 ("高字节1")
                  }
                }
                n2840 = Build Array(w7324, w7322) -> (w7323:i32[])
              }
              frame 8 {
                # "单体电压过低"
                n2841 = disable-structure shown="启用" {
                  disable-tunnel: [w7341 w7344] -> w7336
                  disable-tunnel: [w7339 w7344] -> w7334
                  disable-tunnel: w7333 -> [w7338 _]
                  frame Disabled {
                    n2842 = Unbundle By Name(w7338) -> ("单体电压过低"=w7337:dbl)
                    n2843 = call "输入分辨率计算-EV05.vi"("1字节?"=FALSE, "数值"=w7337, "偏移量"=0.0, "分辨率"=0.001) -> ("低字节"=w7339:dbl, "高字节1"=w7341:dbl)  [unwired: 1 in, 5 out]
                  }
                  frame Enabled {
                    w7344 = 255 ("高字节1")
                  }
                }
                n2844 = Build Array(w7336, w7334) -> (w7335:i32[])
              }
              frame 9 {
                # "充电电流过高"
                n2845 = disable-structure shown="启用" {
                  disable-tunnel: [w7353 w7356] -> w7348
                  disable-tunnel: [w7351 w7356] -> w7346
                  disable-tunnel: w7345 -> [w7350 _]
                  frame Enabled {
                    n2846 = Unbundle By Name(w7350) -> ("充电电流过高"=w7349:dbl)
                    n2847 = call "输入分辨率计算-EV05.vi"("1字节?"=FALSE, "数值"=w7349, "偏移量"=0.0, "分辨率"=0.1) -> ("低字节"=w7351:dbl, "高字节1"=w7353:dbl)  [unwired: 1 in, 5 out]
                  }
                  frame Disabled {
                    w7356 = 255 ("高字节1")
                  }
                }
                n2848 = Build Array(w7348, w7346) -> (w7347:dbl[])
              }
              frame 10 {
                # "放电电流过高"
                n2849 = disable-structure shown="启用" {
                  disable-tunnel: [w7365 w7368] -> w7360
                  disable-tunnel: [w7363 w7368] -> w7358
                  disable-tunnel: w7357 -> [w7362 _]
                  frame Disabled {
                    n2850 = Unbundle By Name(w7362) -> ("放电电流过高"=w7361:dbl)
                    n2851 = call "输入分辨率计算-EV05.vi"("1字节?"=FALSE, "数值"=w7361, "偏移量"=-3000.0, "分辨率"=0.1) -> ("低字节"=w7363:dbl, "高字节1"=w7365:dbl)  [unwired: 1 in, 5 out]
                  }
                  frame Enabled {
                    w7368 = 255 ("高字节1")
                  }
                }
                n2852 = Build Array(w7360, w7358) -> (w7359:i32[])
              }
              frame 11 {
                # "单组温度不均衡"
                n2853 = disable-structure shown="启用" {
                  disable-tunnel: [w7375 255 ("高字节1")] -> w7371
                  disable-tunnel: w7369 -> [w7373 _]
                  frame Disabled {
                    n2854 = Unbundle By Name(w7373) -> ("单组温度不均衡"=w7372:dbl)
                    n2855 = call "输入分辨率计算-EV05.vi"("1字节?"=TRUE, "数值"=w7372, "偏移量"=0.0, "分辨率"=1.0) -> ("高字节1"=w7375:dbl)  [unwired: 1 in, 6 out]
                  }
                  frame Enabled {
                  }
                }
                n2856 = Build Array(w7371) -> (w7370:i32[])
              }
              frame 12 {
                # "SOC过高"
                n2857 = Unbundle By Name(w7383) -> ("SOC过高"=w7382:dbl)
                n2858 = call "输入分辨率计算-EV05.vi"("1字节?"=FALSE, "数值"=w7382, "偏移量"=0.0, "分辨率"=0.1) -> ("低字节"=w7384:dbl, "高字节1"=w7385:dbl)  [unwired: 1 in, 5 out]
                n2859 = call "二进制解析-8.6.vi"("索引"=4, "数值"=w7385) -> ("低位子数组"=w7388:i32[])  [unwired: 3 out]
                n2860 = call "二进制解析-8.6.vi"("索引"=4, "数值"=w7384) -> ("低位子数组"=w7380:i32[], "高位子数组"=w7387:i32[])  [unwired: 2 out]
                n2861 = Insert Into Array(array=w7388, new element=w7387) -> (w7386:i32[])  [unwired: 1 in]
                n2862 = call "数值二进制转十进制-8.6.vi"("子数组"=w7386) -> ("十进制数值"=w7381:i32)  [unwired: 4 out]
                n2863 = disable-structure shown="启用" {
                  disable-tunnel: w7381 -> [w7396 _]
                  disable-tunnel: [w7396 255 ("高字节1")] -> w7379
                  disable-tunnel: [w7395 i32[] [] ("低位子数组 27")] -> _
                  disable-tunnel: w7380 -> [w7395 _]
                  frame Disabled {
                  }
                  frame Enabled {
                  }
                }
                n2864 = Build Array(w7379, w7379) -> (w7392:i32[])
              }
              frame 13 {
                # "SOC过低"
                n2865 = Unbundle By Name(w7404) -> ("SOC过低"=w7403:dbl)
                n2866 = call "输入分辨率计算-EV05.vi"("1字节?"=FALSE, "数值"=w7403, "偏移量"=0.0, "分辨率"=0.1) -> ("低字节"=w7401:dbl, "高字节1"=w7402:dbl)  [unwired: 1 in, 5 out]
                n2867 = call "二进制解析-8.6.vi"("索引"=4, "数值"=w7402) -> ("低位子数组"=w7400:i32[])  [unwired: 3 out]
                n2868 = disable-structure shown="启用" {
                  disable-tunnel: w7401 -> [w7411 _]
                  disable-tunnel: [w7411 255 ("高字节1")] -> w7399
                  disable-tunnel: w7400 -> [w7410 _]
                  disable-tunnel: [w7410 i32[] [] ("低位子数组")] -> _
                  frame Disabled {
                    (unwired) i32[] [] ("低位子数组 4")
                  }
                  frame Enabled {
                  }
                }
                n2869 = Build Array(w7399, w7399) -> (w7407:i32[])
              }
              frame 14 {
                # "内阻过大"
                n2870 = disable-structure shown="启用" {
                  disable-tunnel: w7416 -> [w7421 _]
                  disable-tunnel: [w7417 255 ("高字节1")] -> w7414
                  frame Disabled {
                    n2871 = Unbundle By Name(w7421) -> ("内阻过大"=w7420:dbl)
                    n2872 = call "输入分辨率计算-EV05.vi"("1字节?"=TRUE, "数值"=w7420, "分辨率"=0.1) -> ("高字节1"=w7417:dbl)  [unwired: 2 in, 6 out]
                  }
                  frame Enabled {
                  }
                }
                n2873 = Build Array(w7414) -> (w7415:i32[])
              }
              frame 15 {
                # "极柱温度过高"
                n2874 = disable-structure shown="启用" {
                  disable-tunnel: w7425 -> [w7431 _]
                  disable-tunnel: [w7427 255 ("高字节1")] -> w7423
                  frame Disabled {
                    n2875 = Unbundle By Name(w7431) -> ("极柱温度过高"=w7430:dbl)
                    n2876 = call "输入分辨率计算-EV05.vi"("1字节?"=TRUE, "数值"=w7430, "偏移量"=-40.0, "分辨率"=1.0) -> ("高字节1"=w7427:dbl)  [unwired: 1 in, 6 out]
                  }
                  frame Enabled {
                  }
                }
                n2877 = Build Array(w7423) -> (w7424:i32[])
              }
              frame 16 {
                # "SOH过低"
                n2878 = disable-structure shown="启用" {
                  disable-tunnel: [w7448 w7456] -> w7435
                  disable-tunnel: w7434 -> [w7445 _]
                  disable-tunnel: [w7437 w7456] -> w7433
                  frame Disabled {
                    n2879 = Unbundle By Name(w7445) -> ("SOH过低"=w7444:dbl)
                    n2880 = call "输入分辨率计算-EV05.vi"("1字节?"=FALSE, "数值"=w7444, "偏移量"=0.0, "分辨率"=0.1) -> ("低字节"=w7446:dbl, "高字节1"=w7447:dbl)  [unwired: 1 in, 5 out]
                    n2881 = call "二进制解析-8.6.vi"("索引"=4, "数值"=w7447) -> ("低位子数组"=w7450:i32[])  [unwired: 3 out]
                    n2882 = call "二进制解析-8.6.vi"("索引"=4, "数值"=w7446) -> ("低位子数组"=w7439:i32[], "高位子数组"=w7449:i32[])  [unwired: 2 out]
                    n2883 = call "二进制解析-8.6.vi"("索引"=4, "数值"=0) -> ("低位子数组"=w7440:i32[])  [unwired: 3 out]
                    n2884 = Insert Into Array(array=w7450, new element=w7449) -> (w7443:i32[])  [unwired: 1 in]
                    n2885 = Insert Into Array(array=w7439, new element=w7440) -> (w7438:i32[])  [unwired: 1 in]
                    n2886 = call "数值二进制转十进制-8.6.vi"("子数组"=w7443) -> ("十进制数值"=w7448:i32)  [unwired: 4 out]
                    n2887 = call "数值二进制转十进制-8.6.vi"("子数组"=w7438) -> ("十进制数值"=w7437:i32)  [unwired: 4 out]
                  }
                  frame Enabled {
                    w7456 = 255 ("高字节1")
                  }
                }
                n2888 = Build Array(w7435, w7433) -> (w7436:i32[])
              }
            }
            n2889 = Insert Into Array(array=w7241, new element=w7242) -> (w7240:dbl[])  [unwired: 1 in]
          }
